vi "EM9636B_AD(高速)离线采集数据回放.vi"() -> ()   [LabVIEW 2011]
panel:
  out "是否伪同步":i32
  out "AD物理值":dbl[][](array[numeric])
  out "组频率值":dbl
  out "终止通道":i32
  out "起始通道":i32
  in  "下一批":bool
  in  "上一批":bool
  in  "停止":bool
  in  "读取位置":i32(slide)
  out "实际字节数":u32
  out "波形图":waveform(dbl)[](graph)
  out "通道数量":i32
  out "每组字节数":i32
  out "总数据量（字节）":i32
  out "总数据组数":i32
  in  "每次读取个数":i32=5000 min=10
  out "通道切换频率值":dbl
  out "错误输出":errorcluster
  # "0表示不是伪同步，1为伪同步"
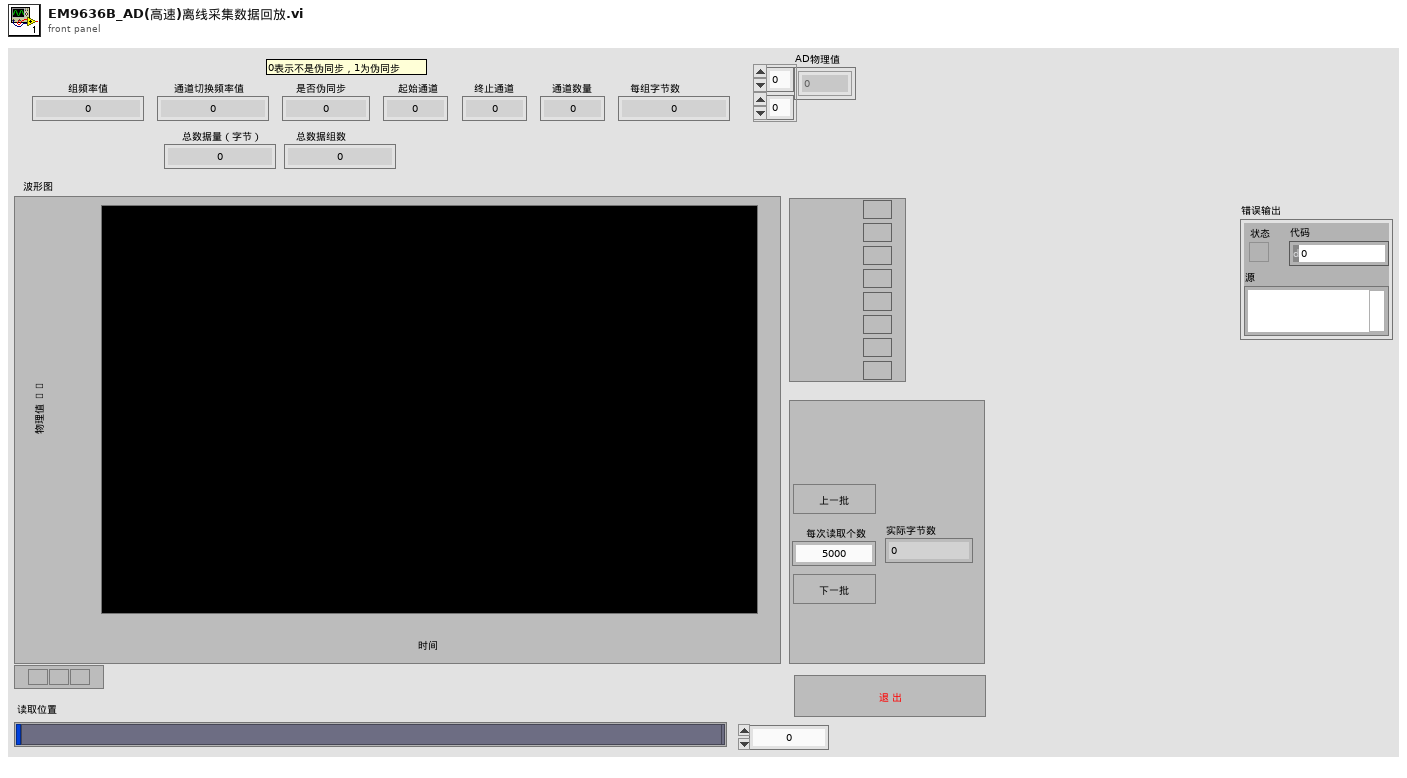
[diagram p1: front panel]
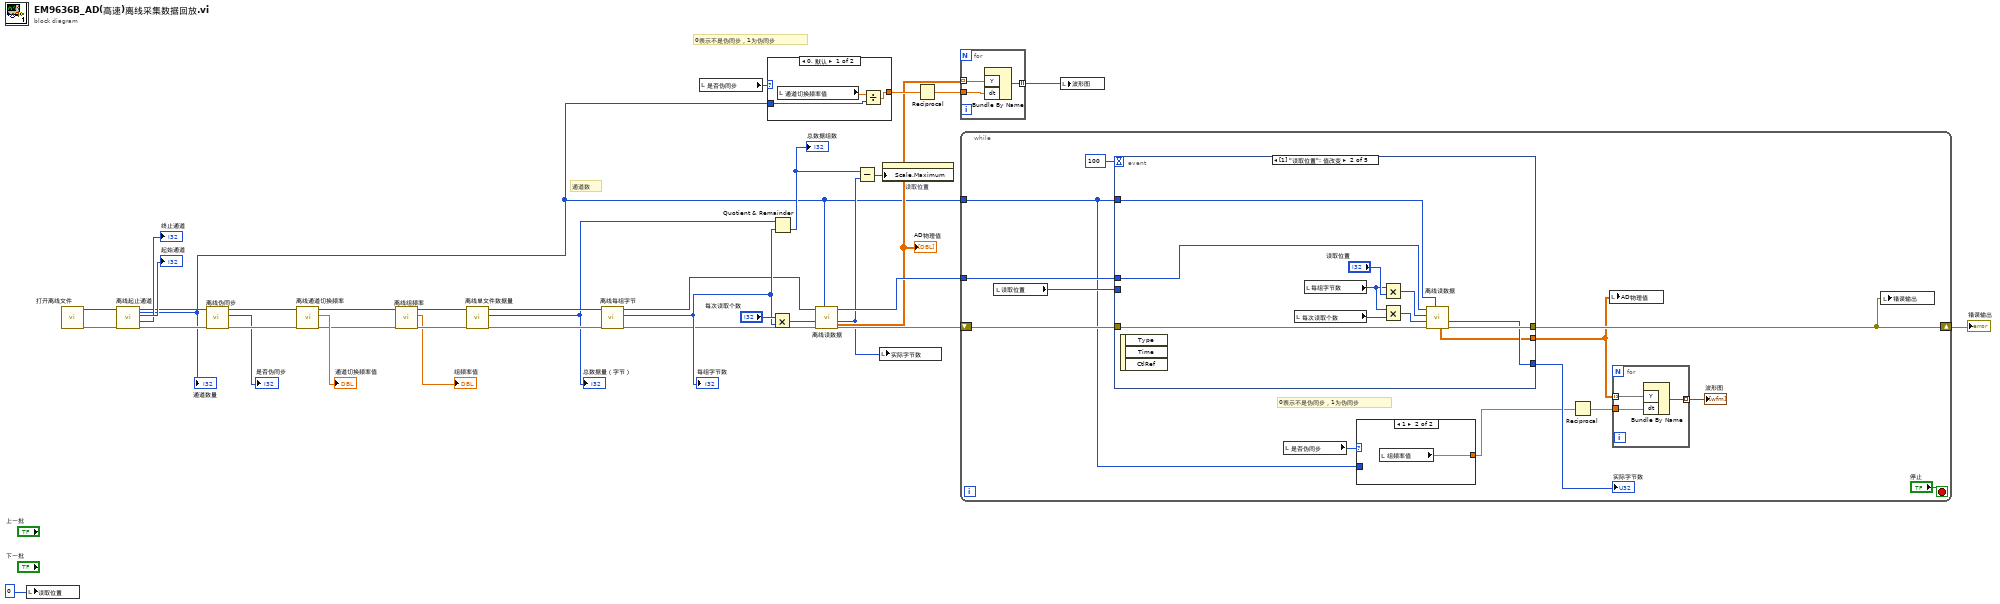
[diagram p0: block diagram]
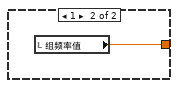
[diagram p2: hidden frame]
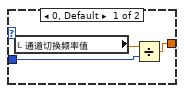
[diagram p3: hidden frame]
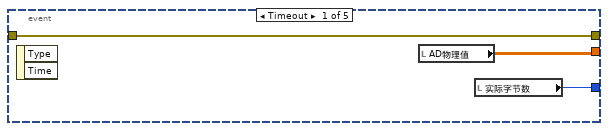
[diagram p4: hidden frame]
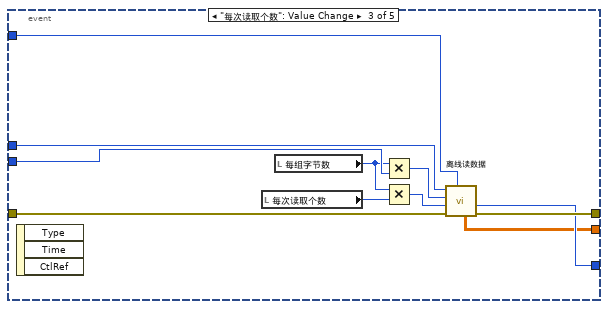
[diagram p5: hidden frame]
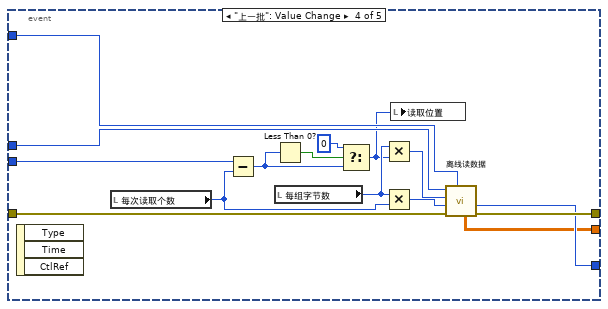
[diagram p6: hidden frame]
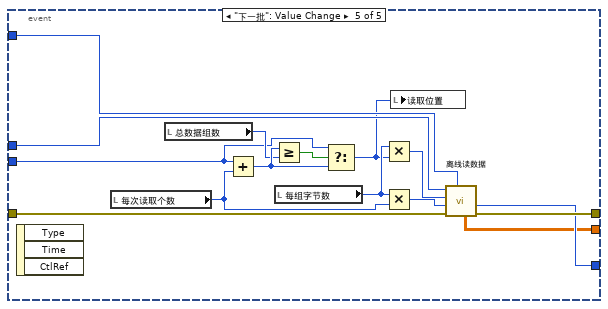
[diagram p7: hidden frame]
diagram:
  # "0表示不是伪同步，1为伪同步"
  # "通道数"
  n1 = local write "读取位置"(0 ("读取位置")) -> ()
  n2 = call "打开离线文件.vi"() -> ("错误输出"=w35:errorcluster, "文件句柄"=w36:i32)  [unwired: 10 in]
  n3 = call "离线起止通道.vi"("错误输入"=w35, "文件句柄"=w36) -> ("错误输出"=w6:errorcluster, "终止通道"=→"终止通道":i32, "起始通道"=→"起始通道":i32, "文件句柄出"=w5:i32, "通道数量"=w1:i32)  [unwired: 5 in]
  "通道数量" <- w1
  n4 = call "离线伪同步.vi"("错误输入"=w6, "文件句柄"=w5) -> ("错误输出"=w7:errorcluster, "是否伪同步"=→"是否伪同步":i32, "文件句柄出"=w4:i32)  [unwired: 7 in]
  n5 = call "离线通道切换频率.vi"("错误输入"=w7, "文件句柄"=w4) -> ("错误输出"=w14:errorcluster, "采集频率"=→"通道切换频率值":dbl, "文件句柄出"=w15:i32)  [unwired: 7 in]
  n6 = call "离线组频率.vi"("错误输入"=w14, "文件句柄"=w15) -> ("错误输出"=w17:errorcluster, "采集频率"=→"组频率值":dbl, "文件句柄出"=w16:i32)  [unwired: 7 in]
  n7 = call "离线单文件数据量.vi"("错误输入"=w17, "文件句柄"=w16) -> ("错误输出"=w32:errorcluster, "总数据量（字节）"=w31:i32, "文件句柄出"=w33:i32)  [unwired: 7 in]
  "总数据量（字节）" <- w31
  n8 = call "离线每组字节.vi"("错误输入"=w32, "文件句柄"=w33) -> ("错误输出"=w27:errorcluster, "每组字节数"=w29:i32, "文件句柄出"=w28:i32)  [unwired: 7 in]
  "每组字节数" <- w29
  n9 = local read "是否伪同步"() -> (w2:i32)
  n10 = case shown="0, 默认" w2 {
    tunnel: [w38 w40] -> w21
    tunnel: w1 -> [w37 _]
    frame 0, Default {
      n11 = local read "通道切换频率值"() -> (w39:dbl)
      n12 = Divide(x=w39, y=w37) -> (x/y=w38:dbl)
    }
    frame 1 {
      n13 = local read "组频率值"() -> (w40:dbl)
    }
  }
  n14 = Multiply(x="每次读取个数", y=w29) -> (x*y=w24:i32)
  n15 = Quotient & Remainder(x=w31, y=w29) -> (floor(x/y)=w10:i32)  [unwired: 1 out]
  "总数据组数" <- w10
  n16 = call "离线读数据.vi"("通道数"=w1, "错误输入"=w27, "读取字节数"=w24, "文件句柄"=w28) -> ("错误输出"=w25:errorcluster, "实际字节数"=w9:u32, "文件句柄出"=w26:i32, "AD物理值"=w11:dbl[][])  [unwired: 3 in, 1 out]
  "AD物理值" <- w11
  n17 = Subtract(x=w10, y=w9) -> (x-y=w8:u32)
  n18 = local write "实际字节数"(w9) -> ()
  n19 = property on="读取位置" class="Slide (严格)"("Scale.Maximum"=w8) -> ()  [unwired: 2 in, 2 out]
  n20 = Reciprocal(x=w21) -> (1/x=w20:dbl)
  n21 = for {
    tunnel: w11 -> [w43] mode=indexing
    tunnel: w20 -> [w42]
    tunnel: [w41] -> w19 mode=indexing
    n22 = Bundle By Name("Y"=w43, "dt"=w42) -> (w41:waveform(dbl))  [unwired: 1 in]
  }
  n23 = while {
    tunnel: w26 -> [w56]
    tunnel: w1 -> [w44]
    shift-right: [w48] -> w22
    shift-left: w25 -> [w55]
    stop <- "停止" stop-if-true
    # "0表示不是伪同步，1为伪同步"
    n24 = local read "读取位置"() -> (w51:i32)
    n25 = event shown="[1] \"读取位置\": 值改变" {
      selector: _ -> [_ _ _ _ _]
      dyn-events: _ -> [_ _ _ _ _]
      timeout: 100 -> [_ _ _ _ _]
      tunnel: w56 -> [_ w77 w88 w103 w118]
      tunnel: w55 -> [w65 w76 w87 w102 w117]
      tunnel: w44 -> [_ w71 w83 w98 w113]
      tunnel: [w64 w67 w78 w89 w104] -> w47
      tunnel: [w66 w74 w85 w100 w115] -> w52
      tunnel: [w65 w75 w86 w101 w116] -> w48
      tunnel: w51 -> [_ _ w82 w95 w105]
      event Timeout {
        n26 = event-data() -> ()  [unwired: 1 in, 2 out]
        n27 = local read "AD物理值"() -> (w64:dbl[][])
        n28 = local read "实际字节数"() -> (w66:u32)
      }
      event "读取位置": Value Change {
        n29 = event-data() -> ()  [unwired: 1 in, 3 out]
        n30 = local read "每次读取个数"() -> (w69:i32)
        n31 = local read "每组字节数"() -> (w70:i32)
        n32 = Multiply(x=w70, y="读取位置") -> (x*y=w72:i32)
        n33 = Multiply(x=w70, y=w69) -> (x*y=w68:i32)
        n34 = call "离线读数据.vi"("通道数"=w71, "错误输入"=w76, "读取字节数"=w68, "读取位置"=w72, "文件句柄"=w77) -> ("错误输出"=w75:errorcluster, "实际字节数"=w74:u32, "AD物理值"=w67:dbl[][])  [unwired: 2 in, 2 out]
      }
      event "每次读取个数": Value Change {
        n35 = event-data() -> ()  [unwired: 1 in, 3 out]
        n36 = local read "每次读取个数"() -> (w79:i32)
        n37 = local read "每组字节数"() -> (w80:i32)
        n38 = Multiply(x=w80, y=w82) -> (x*y=w84:i32)
        n39 = Multiply(x=w80, y=w79) -> (x*y=w81:i32)
        n40 = call "离线读数据.vi"("通道数"=w83, "错误输入"=w87, "读取字节数"=w81, "读取位置"=w84, "文件句柄"=w88) -> ("错误输出"=w86:errorcluster, "实际字节数"=w85:u32, "AD物理值"=w78:dbl[][])  [unwired: 2 in, 2 out]
      }
      event "上一批": Value Change {
        n41 = event-data() -> ()  [unwired: 1 in, 3 out]
        n42 = local read "每次读取个数"() -> (w94:i32)
        n43 = Subtract(x=w95, y=w94) -> (x-y=w92:i32)
        n44 = Less Than 0?(x=w92) -> (x < 0?=w93:bool)
        n45 = local read "每组字节数"() -> (w96:i32)
        n46 = Select(t=0, s=w93, f=w92) -> (s? t:f=w90:i32)
        n47 = Multiply(x=w96, y=w90) -> (x*y=w99:i32)
        n48 = Multiply(x=w96, y=w94) -> (x*y=w97:i32)
        n49 = local write "读取位置"(w90) -> ()
        n50 = call "离线读数据.vi"("通道数"=w98, "错误输入"=w102, "读取字节数"=w97, "读取位置"=w99, "文件句柄"=w103) -> ("错误输出"=w101:errorcluster, "实际字节数"=w100:u32, "AD物理值"=w89:dbl[][])  [unwired: 2 in, 2 out]
      }
      event "下一批": Value Change {
        n51 = event-data() -> ()  [unwired: 1 in, 3 out]
        n52 = local read "每次读取个数"() -> (w110:i32)
        n53 = local read "总数据组数"() -> (w106:i32)
        n54 = Add(x=w105, y=w110) -> (x+y=w107:i32)
        n55 = Greater Or Equal?(x=w107, y=w106) -> (x >= y?=w109:bool)
        n56 = local read "每组字节数"() -> (w111:i32)
        n57 = Select(t=w105, s=w109, f=w107) -> (s? t:f=w108:i32)
        n58 = Multiply(x=w111, y=w108) -> (x*y=w114:i32)
        n59 = Multiply(x=w111, y=w110) -> (x*y=w112:i32)
        n60 = local write "读取位置"(w108) -> ()
        n61 = call "离线读数据.vi"("通道数"=w113, "错误输入"=w117, "读取字节数"=w112, "读取位置"=w114, "文件句柄"=w118) -> ("错误输出"=w116:errorcluster, "实际字节数"=w115:u32, "AD物理值"=w104:dbl[][])  [unwired: 2 in, 2 out]
      }
    }
    "实际字节数" <- w52
    n62 = local read "是否伪同步"() -> (w46:i32)
    n63 = case shown="1" w46 {
      tunnel: [w58 w60] -> w45
      tunnel: w44 -> [w57 _]
      frame 0, Default {
        n64 = local read "通道切换频率值"() -> (w59:dbl)
        n65 = Divide(x=w59, y=w57) -> (x/y=w58:dbl)
      }
      frame 1 {
        n66 = local read "组频率值"() -> (w60:dbl)
      }
    }
    n67 = Reciprocal(x=w45) -> (1/x=w50:dbl)
    n68 = local write "AD物理值"(w47) -> ()
    n69 = for {
      tunnel: w47 -> [w63] mode=indexing
      tunnel: w50 -> [w62]
      tunnel: [w61] -> w49 mode=indexing
      n70 = Bundle By Name("Y"=w63, "dt"=w62) -> (w61:waveform(dbl))  [unwired: 1 in]
    }
    "波形图" <- w49
    n71 = local write "错误输出"(w48) -> ()
  }
  "错误输出" <- w22
  n72 = local write "波形图"(w19) -> ()
